vi "Robot_Targeting_adjustment.vi"() -> ()   [LabVIEW 2018]
uses:
  <vilib>/Rock Robotics/Network Tables/NT Read Number.vi
  <vilib>/addons/control/pid/pid.llb/PID (DBL).vi
  <vilib>/addons/control/pid/NI_PID_pid.lvlib
panel:
  in  "Tape Strafe":T1={"proportional gain (Kc)"=0.035, "integral time (Ti, min)"=0.0, "derivative time (Td, min)"=0.0018} {"derivative time (Td, min)" format="%.3f"; "integral time (Ti, min)" format="%.3f"; "proportional gain (Kc)" format="%.3f"}
  in  "Tape Range":cluster{"output high":dbl, "output low":dbl}={"output high"=0.7, "output low"=-0.7} {"output low" format="%.2f"; "output high" format="%.2f"}
  # ".7\n-.7"
  # "1\n-1"
  # ".5\n-.5"
  # "Rotation"
  # "Strafe"
  # "Forward back"
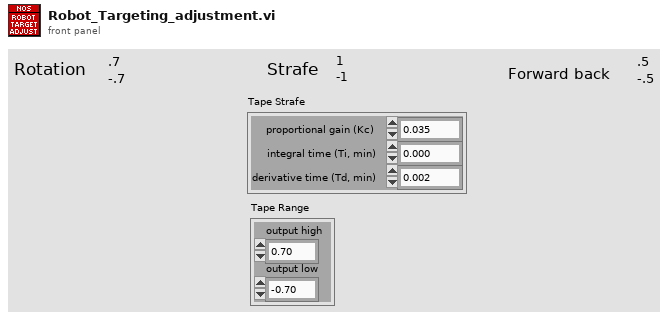
[diagram p1: front panel]
types:
  T1 = cluster{"proportional gain (Kc)":dbl, "integral time (Ti, min)":dbl, "derivative time (Td, min)":dbl}
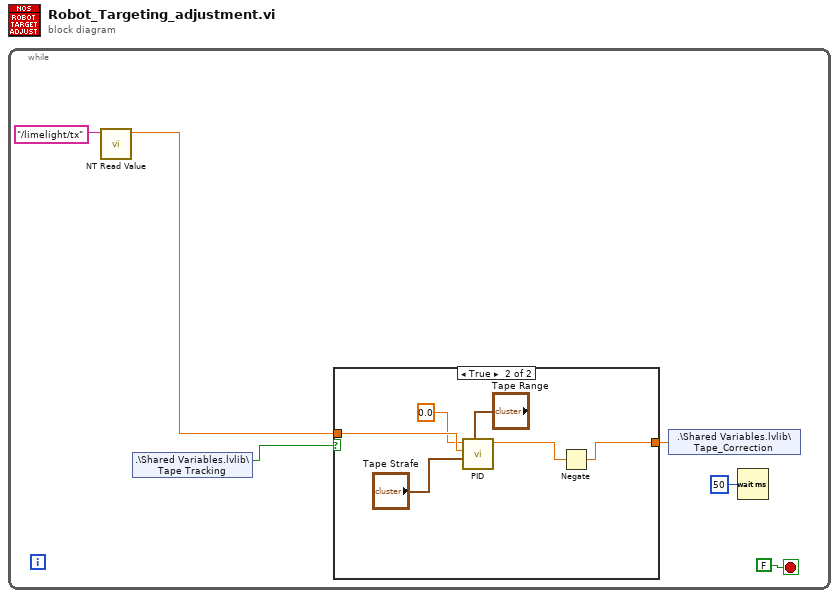
[diagram p0: block diagram]
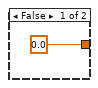
[diagram p2: hidden frame]
diagram:
  n1 = while {
    stop <- FALSE stop-if-true
    n2 = call-poly <vilib>:"NT Read Value.vi"("Name"="/limelight/tx") -> ("Numeric"=w4:dbl)  [unwired: 9 in, 1 out]
    n3 = shared-variable ".\\Shared Variables.lvlib\\Tape Tracking"() -> (w3:bool)  [unwired: 1 in, 1 out]
    n4 = case shown="True" w3 {
      tunnel: w4 -> [_ w11]
      tunnel: [0.0 ("output") w8] -> w2
      frame False {
      }
      frame True {
        n5 = call-poly <vilib>:"PID.vi"("output range"="Tape Range", "PID gains"="Tape Strafe", "process variable"=w11, "setpoint"=0.0) -> ("output"=w9:dbl)  [unwired: 6 in, 1 out]
        n6 = Negate(x=w9) -> (-x=w8:dbl)
      }
    }
    n7 = shared-variable ".\\Shared Variables.lvlib\\Tape_Correction"(w2) -> ()  [unwired: 1 in, 1 out]
    n8 = Wait (ms)(milliseconds to wait=u32 50) -> ()  [unwired: 1 out]
  }
